vi "LinearSystemLoop_SetNextR.vi"(9 "R":T3, 11 "input inear System Loop":T1) -> (0 "Size Coerced":bool, 3 "out Linear System Loop":T1)   [LabVIEW 2019, in "Trajectory_Library.lvlib"]
doc: "Set the next reference r.\n \nInputs:\n - LinearSystemLoop -- system data cluster\n - nextR -- Next reference.\n\nOutputs:\n - outLinearSystemLoop -- updated system data cluster\n - sizeCoerced -- If TRUE, an error occured."
uses:
  Trajectory_Library.lvlib
  TypeDef/LINEAR_SYSTEM_LOOP.ctl
  TypeDef/LINEAR_QUADRATIC_REGULATOR.ctl
  <vilib>/Analysis/Matrix/Datatypes/RealMatrix.ctl
  TypeDef/LINEAR_PLANT_INV_FF.ctl
  TypeDef/KALMAN_FILTER.ctl
  TypeDef/LINEAR_SYSTEM.ctl
  MatBuilder_Create.vi
  <vilib>/Analysis/Matrix/NI_Matrix.lvlib
panel:
  # "<States,1>"
  # "<FUTURE --- CLAMP TYPE -- For now\nuse Normalize>"
  # "Steady State Gain  \n<States,Outputs>"
  # "State Estimate <Statess,1>"
  # "<States,States>"
  # "<States,Inputs>"
  # "<Outputs,States>"
  # "<Outputs,Inputs>"
  # "<States,1>"
  # "<Inputs,1>"
  # "<States,Inputs>"
  # "<States,States>"
  # "Ref State <States,1>"
  # "Comp and capped \noutput <Inputs,1>"
  # "Controller gain\n<Inputs,States>"
  # "<States,1>"
  # "<FUTURE --- CLAMP TYPE -- For now\nuse Normalize>"
  # "Steady State Gain  \n<States,Outputs>"
  # "State Estimate <Statess,1>"
  # "<States,States>"
  # "<States,Inputs>"
  # "<Outputs,States>"
  # "<Outputs,Inputs>"
  # "<States,1>"
  # "<Inputs,1>"
  # "<States,Inputs>"
  # "<States,States>"
  # "Ref State <States,1>"
  # "Comp and capped \noutput <Inputs,1>"
  # "Controller gain\n<Inputs,States>"
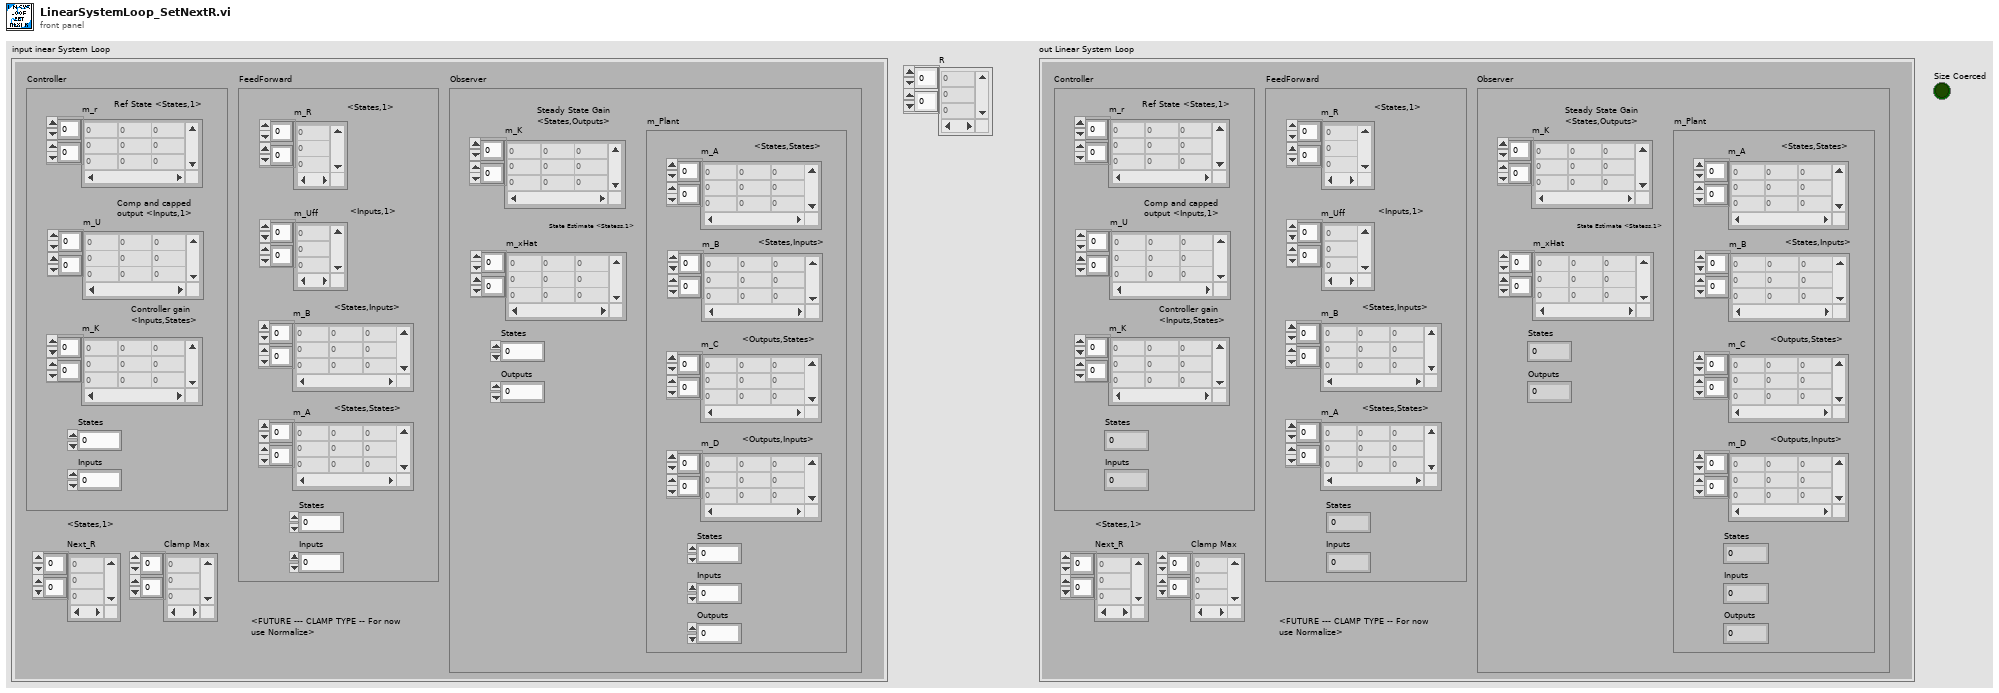
[diagram p1: front panel]
types:
  T1 = typedef "Trajectory_Library.lvlib/LINEAR_SYSTEM_LOOP.ctl" = cluster{"Controller":T2, "FeedForward":T4, "Observer":T5, "Next_R":T3, "Clamp Max":T3}
  T2 = typedef "Trajectory_Library.lvlib/LINEAR_QUADRATIC_REGULATOR.ctl" = cluster{"m_r":T3, "m_U":T3, "m_K":T3, "States":i32, "Inputs":i32}
  T3 = typedef "NI_Matrix.lvlib/RealMatrix.ctl" = dbl[][]
  T4 = typedef "Trajectory_Library.lvlib/LINEAR_PLANT_INV_FF.ctl" = cluster{"m_R":T3, "m_Uff":T3, "m_B":T3, "m_A":T3, "States":i32, "Inputs":i32}
  T5 = typedef "Trajectory_Library.lvlib/KALMAN_FILTER.ctl" = cluster{"m_K":T3, "m_xHat":T3, "States":i32, "Outputs":i32, "m_Plant":T6}
  T6 = typedef "Trajectory_Library.lvlib/LINEAR_SYSTEM.ctl" = cluster{"m_A":T3, "m_B":T3, "m_C":T3, "m_D":T3, "States":i32, "Inputs":i32, "Outputs":i32}
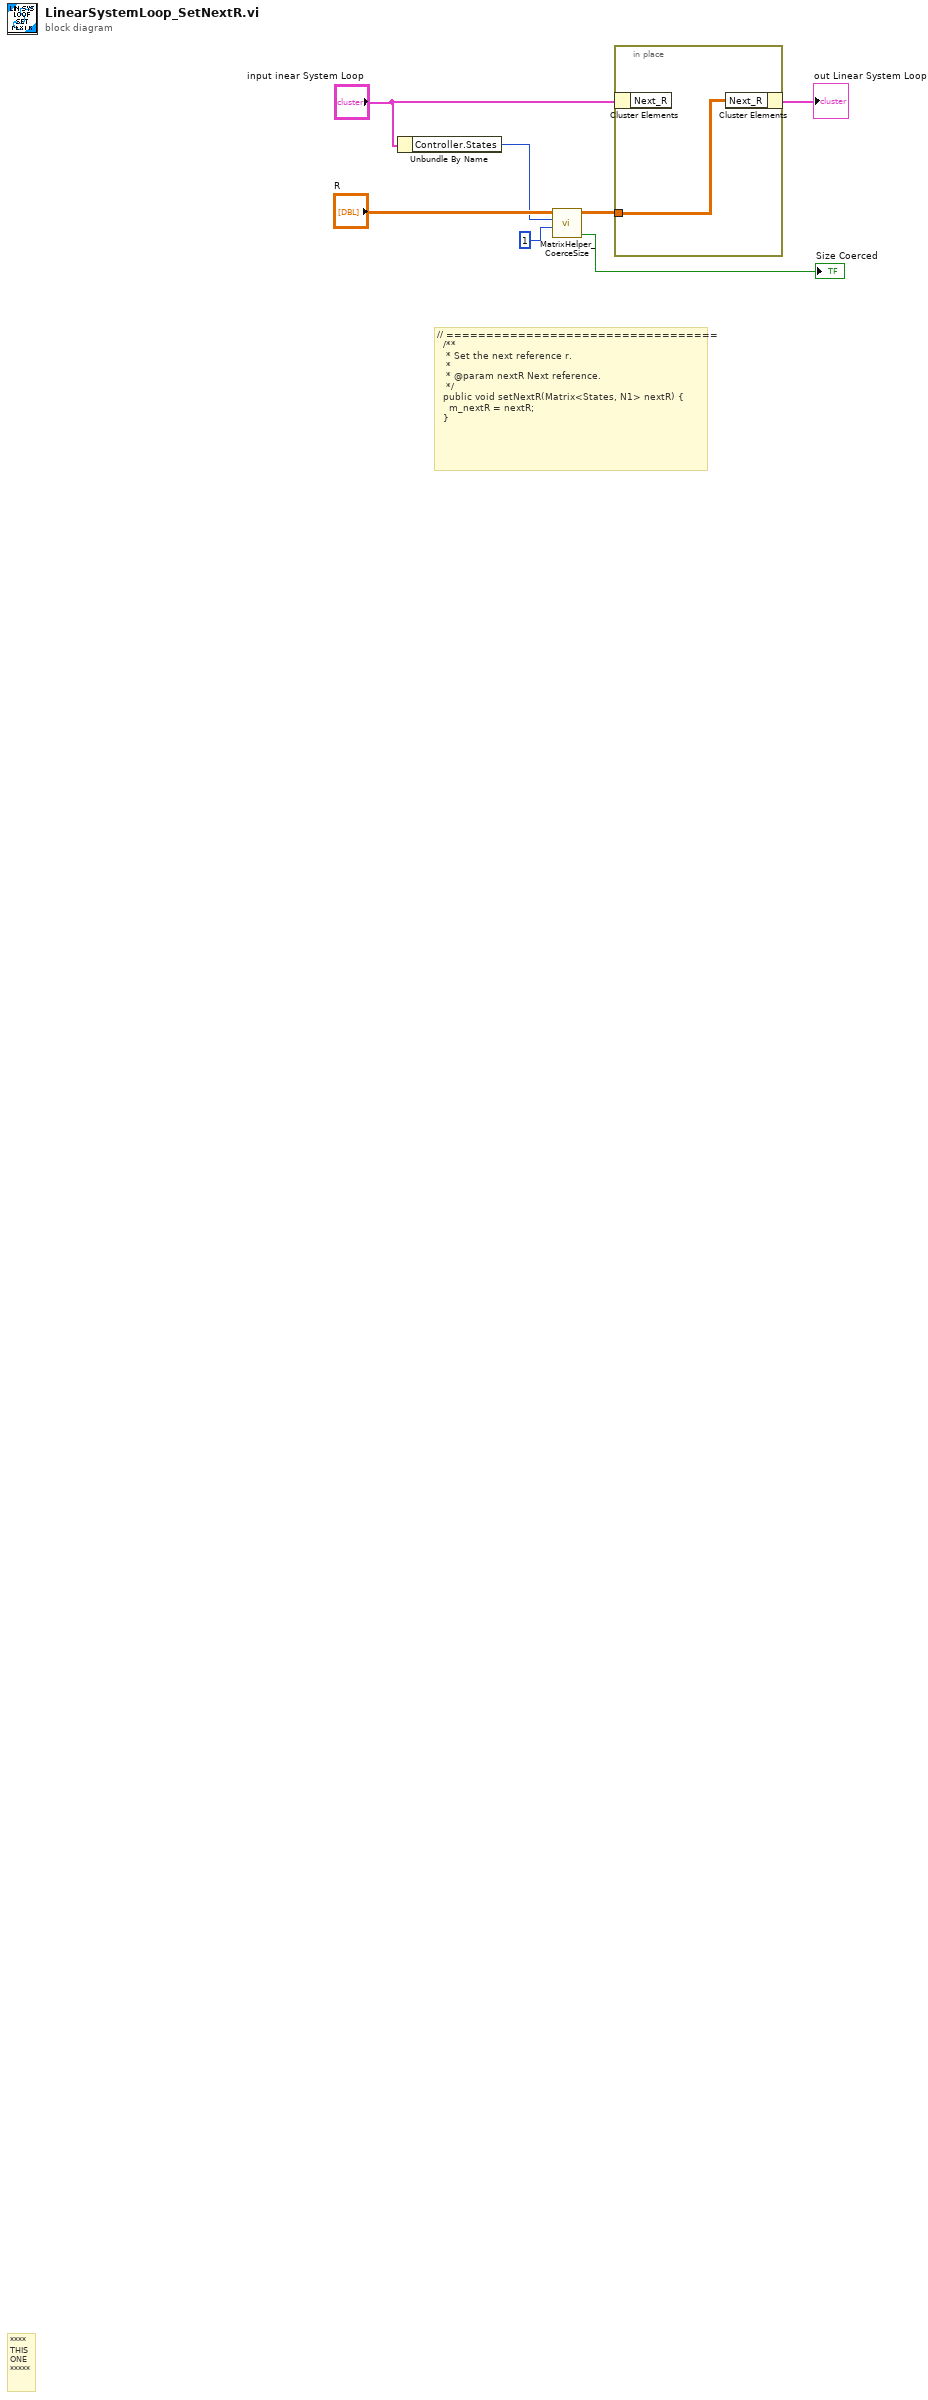
[diagram p0: block diagram]
diagram:
  # "// ==================================\n  /**\n   * Set the next reference r.\n   *\n   * @param nextR Next reference.\n   */\n  public void setNextR(Matrix<States, N1> nextR) {\n    m_nextR = nextR;\n  }"
  # "****\nTHIS\nONE\n*****"
  n1 = Unbundle By Name("input inear System Loop") -> ("Controller.States"=w3:i32)
  n2 = call "MatrixHelper_CoerceSize.vi"("Columns"=1, "Rows"=w3, "input matrix"="R") -> ("Coerced"=→"Size Coerced":bool, "output matrix"=w2:T3)  [unwired: 7 in]
  n3 = in-place {
    in-place-border: w2 -> [w8]
    n4 = in-place-cluster #1("input inear System Loop") -> ()  [unwired: 1 out]
    n5 = in-place-cluster #1("Next_R"=w8) -> (→"out Linear System Loop":T1)
  }
